vi "Get ni_xnet_can_bm_api_ResetStreamingFilterReply.vi"(8 "error in (no error)":errorcluster, 11 "gRPCid":T1) -> (0 "error out":errorcluster, 2 "package_templatemessage":T2, 3 "gRPCid out":T1)   [LabVIEW 2025, in "xnet_can_bus_monitor_api_server.lvlib"]
uses:
  xnet_can_bus_monitor_api_server.lvlib
  2ed25e12-861d-4677-8ead-ace2906b2041.vi
  ni_xnet_can_bm_api_DirectionFilter.ctl
  ni_xnet_can_bm_api_FrameFilter.ctl
  ni_xnet_can_bm_api_FilterInfo.ctl
  ni_xnet_can_bm_api_ErrorInfo.ctl
  ni_xnet_can_bm_api_ResetStreamingFilterReply.ctl
  ni_xnet_can_bm_api_FilterInfo_Flat.ctl
  ni_xnet_can_bm_api_ErrorInfo_Flat.ctl
  ni_xnet_can_bm_api_ResetStreamingFilterReply_Flat.ctl
  <vilib>/gRPC/LabVIEW gRPC Library/Shared/grpcId.ctl
  <vilib>/gRPC/LabVIEW gRPC Library/grpc-lvsupport-release.lvlib
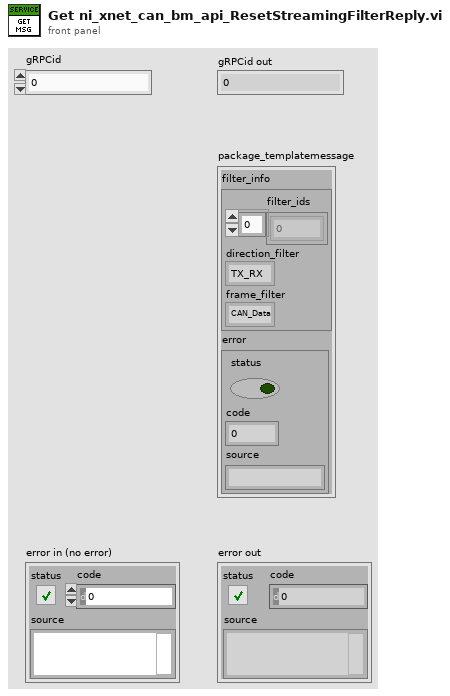
[diagram p1: front panel]
types:
  T1 = typedef "grpc-lvsupport-release.lvlib/grpcId.ctl" = u64
  T2 = typedef "xnet_can_bus_monitor_api_server.lvlib/ni_xnet_can_bm_api_ResetStreamingFilterReply.ctl" = cluster{"filter_info":T3, "error":T6}
  T3 = typedef "xnet_can_bus_monitor_api_server.lvlib/ni_xnet_can_bm_api_FilterInfo.ctl" = cluster{"filter_ids":u32[], "direction_filter":T4, "frame_filter":T5}
  T4 = typedef "xnet_can_bus_monitor_api_server.lvlib/ni_xnet_can_bm_api_DirectionFilter.ctl" = enum32{"TX_RX", "RX", "TX"}
  T5 = typedef "xnet_can_bus_monitor_api_server.lvlib/ni_xnet_can_bm_api_FrameFilter.ctl" = enum32{"CAN_Data", "CAN_Remote", "CAN_Bus_Error", "CAN_2_Data", "CAN_FD_Data", "CAN_FD_BRS_Data", "J1939_Data", "Delay", "Log_Trigger", "Start_Trigger", "All"}
  T6 = typedef "xnet_can_bus_monitor_api_server.lvlib/ni_xnet_can_bm_api_ErrorInfo.ctl" = errorcluster
  T7 = typedef "xnet_can_bus_monitor_api_server.lvlib/ni_xnet_can_bm_api_ResetStreamingFilterReply_Flat.ctl" = cluster{"filter_info":T8, "error":T9}
  T8 = typedef "xnet_can_bus_monitor_api_server.lvlib/ni_xnet_can_bm_api_FilterInfo_Flat.ctl" = cluster{"filter_ids":u32[], "direction_filter":T4, "frame_filter":T5}
  T9 = typedef "xnet_can_bus_monitor_api_server.lvlib/ni_xnet_can_bm_api_ErrorInfo_Flat.ctl" = errorcluster
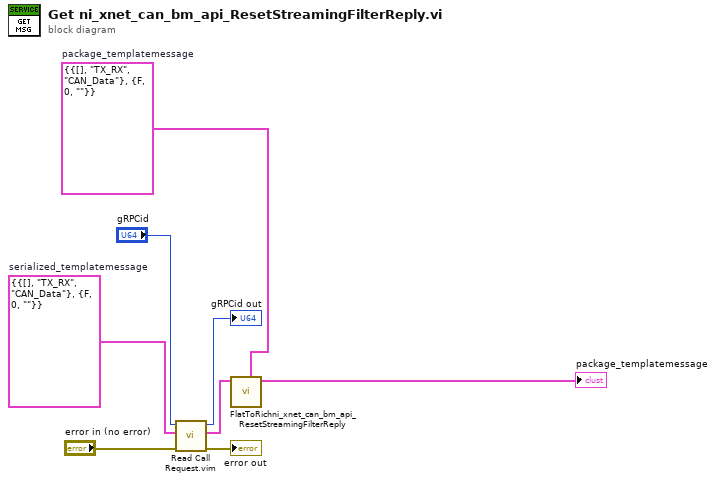
[diagram p0: block diagram]
diagram:
  w6 = T7 {"filter_info"={"filter_ids"=[], "direction_filter"=enum."TX_RX", "frame_filter"=enum."CAN_Data"}, "error"={"status"=FALSE, "code"=0, "source"=""}}  # serialized_templatemessage
  w5 = T2 {"filter_info"={"filter_ids"=[], "direction_filter"=enum."TX_RX", "frame_filter"=enum."CAN_Data"}, "error"={"status"=FALSE, "code"=0, "source"=""}}  # package_templatemessage
  n1 = call "Read Call Request.vim"("error in"="error in (no error)", "Request Type"=w6, "gRPCid in"="gRPCid") -> ("error out"=→"error out":errorcluster, "Request Data"=w4:T7, "gRPCid out"=→"gRPCid out":T1)  [unwired: 6 in]
  n2 = call "FlatToRichni_xnet_can_bm_api_ResetStreamingFilterReply.vi"("OutputClusterType"=w5, "InputCluster"=w4) -> ("OutputCluster"=→"package_templatemessage":T2)  [unwired: 9 in]
